vi "Setup DMM to Acquire Multiple Samples.vi"(8 "error in (no error)":errorcluster, 10 "DMM Parameters":T1={"Function"=enum."DC Volts", "Resolution in Digits"=5.5, "Range"=0.02, "Trigger Source"=enum."Immediate", "Trigger Delay (sec)"=-1.0, "Trigger Count"=1, "Sample Count"=1, "Sample Trigger"=enum."Immediate", "Sample Interval (sec)"=-1.0, "Trigger Slope"=enum."Falling Edge", "Sample Trigger Slope"=enum."Falling Edge"} {"Sample Count" format="%.2f"; "Range" format="%.2f"; "Resolution in Digits" items=["3 1/2"=3.5, "4 1/2"=4.5, "5 1/2"=5.5, "6 1/2"=6.5, "7 1/2"=7.5]}, 11 "instrument handle":refnum<k15>) -> (0 "error out":errorcluster, 3 "instrument handle out":refnum<k15>)   [LabVIEW 2021, in "PMIC Common.lvlib"]
uses:
  PMIC Common.lvlib
  DMM Parameters.ctl
  <instrlib>/niDMM/nidmm.llb/niDMM Function.ctl
  <instrlib>/niDMM/nidmm.llb/niDMM Resolution in Digits.ctl
  <instrlib>/niDMM/nidmm.llb/niDMM Configure Measurement Digits.vi
  <instrlib>/niDMM/nidmm.llb/niDMM Sample Trigger.ctl
  <instrlib>/niDMM/nidmm.llb/niDMM Trigger.ctl
  <instrlib>/niDMM/nidmm.llb/niDMM Slope.ctl
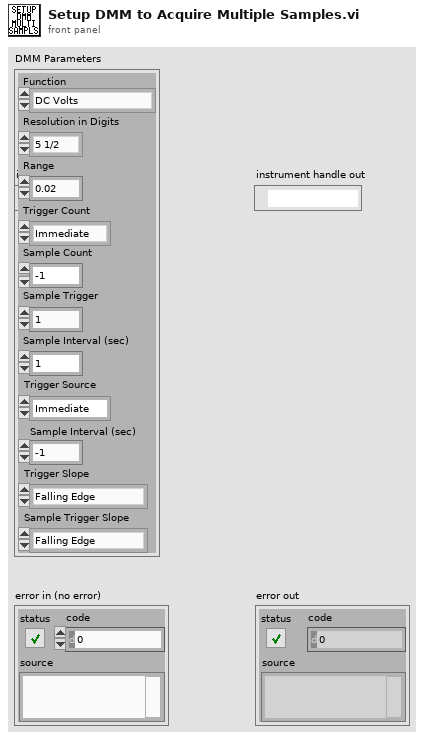
[diagram p1: front panel]
types:
  T1 = typedef "PMIC Common.lvlib/DMM Parameters.ctl" = cluster{"Function":T2, "Resolution in Digits":T3, "Range":dbl, "Trigger Source":T4, "Trigger Delay (sec)":dbl, "Trigger Count":i32, "Sample Count":i32, "Sample Trigger":T5, "Sample Interval (sec)":dbl, "Trigger Slope":T6, "Sample Trigger Slope":T6}
  T2 = typedef "niDMM Function.ctl" = enum16{"DC Volts", "AC Volts", "DC Current", "AC Current", "2-wire Resistance", "4-wire Resistance", "Diode", "Frequency", "Period", "AC Volts DC Coupled", "Capacitance", "Inductance", "Temperature"}
  T3 = typedef "niDMM Resolution in Digits.ctl" = dbl
  T4 = typedef "niDMM Trigger.ctl" = enum16{"Immediate", "External", "TTL 0", "TTL 1", "TTL 2", "TTL 3", "TTL 4", "TTL 5", "TTL 6", "Software", "TTL 7", "PXI Star", "LBR Trig 1", "Aux Trig 1"}
  T5 = typedef "niDMM Sample Trigger.ctl" = enum16{"Immediate", "External", "TTL 0", "TTL 1", "TTL 2", "TTL 3", "TTL 4", "TTL 5", "TTL 6", "Interval", "Software", "TTL 7", "PXI Star", "LBR Trig 1", "Aux Trig 1"}
  T6 = typedef "niDMM Slope.ctl" = enum16{"Rising Edge", "Falling Edge"}
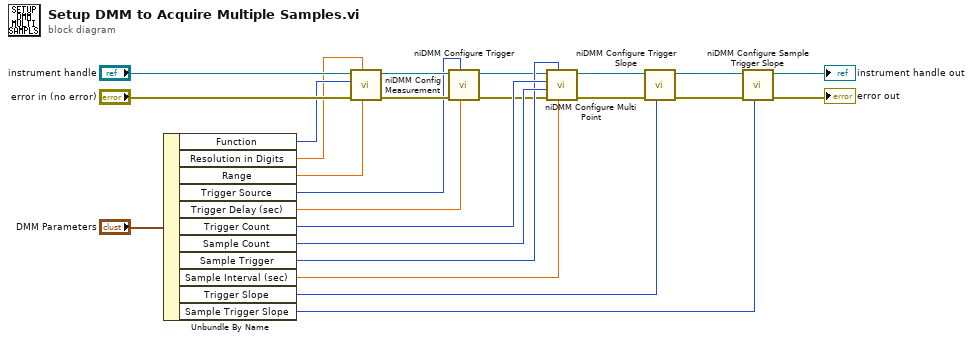
[diagram p0: block diagram]
diagram:
  n1 = Unbundle By Name("DMM Parameters") -> ("Function"=w21:T2, "Resolution in Digits"=w20:T3, "Range"=w19:dbl, "Trigger Source"=w2:T4, "Trigger Delay (sec)"=w1:dbl, "Trigger Count"=w18:i32, "Sample Count"=w17:i32, "Sample Trigger"=w16:T5, "Sample Interval (sec)"=w15:dbl, "Trigger Slope"=w10:T6, "Sample Trigger Slope"=w9:T6)
  n2 = call-poly <instrlib>:"niDMM Config Measurement.vi"("Range"=w19, "Resolution in Digits"=w20, "error in (no error)"="error in (no error)", "Function"=w21, "instrument handle"="instrument handle") -> ("error out"=w7:errorcluster, "instrument handle out"=w8:refnum<k15>)  [unwired: 5 in]
  n3 = call <instrlib>:"niDMM Configure Trigger.vi"("Trigger Delay (sec)"=w1, "Trigger Source"=w2, "error in (no error)"=w7, "instrument handle"=w8) -> ("error out"=w5:errorcluster, "instrument handle out"=w6:refnum<k15>)  [unwired: 6 in]
  n4 = call <instrlib>:"niDMM Configure Multi Point.vi"("Sample Interval (sec)"=w15, "Sample Trigger"=w16, "error in (no error)"=w5, "Sample Count"=w17, "Trigger Count"=w18, "instrument handle"=w6) -> ("error out"=w4:errorcluster, "instrument handle out"=w3:refnum<k15>)  [unwired: 4 in]
  n5 = call <instrlib>:"niDMM Configure Trigger Slope.vi"("Slope"=w10, "error in (no error)"=w4, "instrument handle"=w3) -> ("error out"=w13:errorcluster, "instrument handle out"=w14:refnum<k15>)  [unwired: 7 in]
  n6 = call <instrlib>:"niDMM Configure Sample Trigger Slope.vi"("Slope"=w9, "error in (no error)"=w13, "instrument handle"=w14) -> ("error out"=→"error out":errorcluster, "instrument handle out"=→"instrument handle out":refnum<k15>)  [unwired: 7 in]
